vi "Gear.vi"(11 "Gear Angle State":dbl) -> (0 "LED State":dbl, 3 "Gear Angle Speed":dbl)   [LabVIEW 2016]
uses:
  Joystick Values.vi
  Robot Global Data.vi
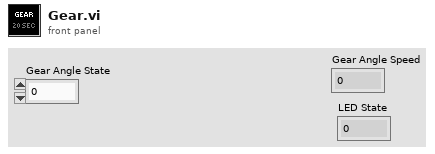
[diagram p1: front panel]
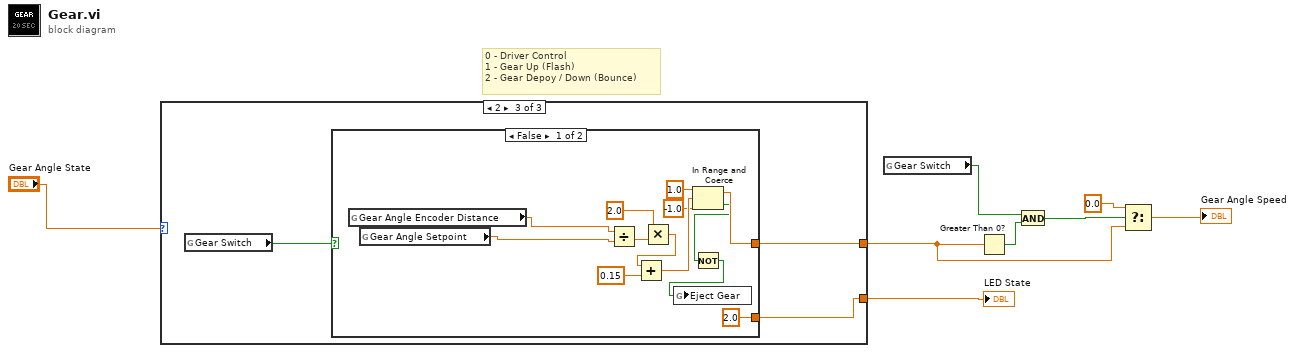
[diagram p0: block diagram]
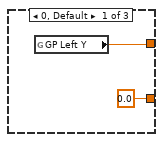
[diagram p2: hidden frame]
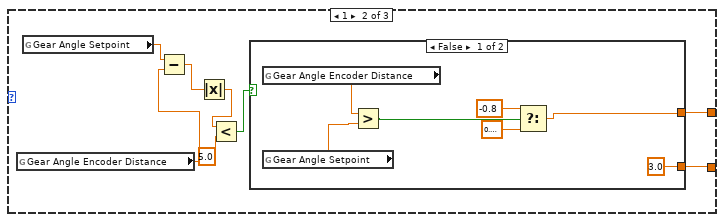
[diagram p3: hidden frame]
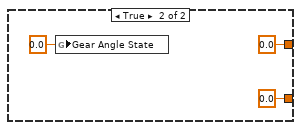
[diagram p4: hidden frame]
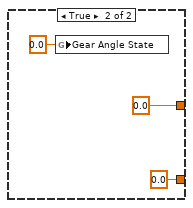
[diagram p5: hidden frame]
diagram:
  # "0 - Driver Control\n1 - Gear Up (Flash)\n2 - Gear Depoy / Down (Bounce)"
  n1 = case shown="2" "Gear Angle State" {
    tunnel: [w10 w18 w31] -> w5
    tunnel: [0.0 ("LED State") w11 w29] -> w2
    frame 0, Default {
      n2 = global read "Joystick Values.vi" "GP Left Y"() -> (w10:dbl)
    }
    frame 1 {
      n3 = global read "Robot Global Data.vi" "Gear Angle Encoder Distance"() -> (w15:dbl)
      n4 = global read "Robot Global Data.vi" "Gear Angle Setpoint"() -> (w16:dbl)
      n5 = Subtract(x=w16, y=w15) -> (x-y=w17:dbl)
      n6 = Absolute Value(x=w17) -> (abs(x)=w14:dbl)
      n7 = Less?(x=w14, y=5.0) -> (x < y?=w12:bool)
      n8 = case shown="False" w12 {
        tunnel: [w23 0.0 ("f")] -> w18
        tunnel: [3.0 ("LED State") 0.0 ("LED State")] -> w11
        frame False {
          n9 = global read "Robot Global Data.vi" "Gear Angle Encoder Distance"() -> (w21:dbl)
          n10 = global read "Robot Global Data.vi" "Gear Angle Setpoint"() -> (w20:dbl)
          n11 = Greater?(x=w21, y=w20) -> (0:w22:bool)
          n12 = Select(t=-0.8, s=w22, f=0.7999999999999999) -> (s? t:f=w23:dbl)
        }
        frame True {
          n13 = global write "Robot Global Data.vi" "Gear Angle State"(0.0 ("Gear Angle State")) -> ()
        }
      }
    }
    frame 2 {
      n14 = global read "Robot Global Data.vi" "Gear Switch"() -> (w30:bool)
      n15 = case shown="False" w30 {
        tunnel: [w37 0.0] -> w31
        tunnel: [2.0 ("LED State") 0.0 ("LED State")] -> w29
        frame False {
          n16 = global read "Robot Global Data.vi" "Gear Angle Encoder Distance"() -> (w43:dbl)
          n17 = global read "Robot Global Data.vi" "Gear Angle Setpoint"() -> (w42:dbl)
          n18 = Divide(x=w43, y=w42) -> (x/y=w41:dbl)
          n19 = Multiply(x=2.0, y=w41) -> (x*y=w39:dbl)
          n20 = Add(x=w39, y=0.15) -> (x+y=w38:dbl)
          n21 = In Range and Coerce(upper limit=1.0, x=w38, lower limit=-1.0) -> (coerced(x)=w37:dbl, In Range?=w34:bool)
          n22 = Not(x=w34) -> (.not. x?=w33:bool)
          n23 = global write "Robot Global Data.vi" "Eject Gear"(w33) -> ()
        }
        frame True {
          n24 = global write "Robot Global Data.vi" "Gear Angle State"(0.0 ("Gear Angle State")) -> ()
        }
      }
    }
  }
  "LED State" <- w2
  n25 = global read "Robot Global Data.vi" "Gear Switch"() -> (w1:bool)
  n26 = Greater Than 0?(x=w5) -> (x > 0?=w6:bool)
  n27 = And(x=w1, y=w6) -> (x .and. y?=w8:bool)
  n28 = Select(t=0.0, s=w8, f=w5) -> (s? t:f=→"Gear Angle Speed":dbl)
